vi "testAESEncryptDecrypt-ECB-256.vi"(8 "error in (no error)":errorcluster, 11 "TestCase in":refnum<class "TestAES.lvclass">) -> (0 "error out":errorcluster, 3 "TestCase out":refnum<class "TestAES.lvclass">)   [LabVIEW 2021, in "TestAES.lvclass"]
uses:
  TestAES.lvclass
  C:/Program Files (x86)/National Instruments/LabVIEW 2021/vi.lib/addons/_JKI Toolkits/VI Tester/TestCase.llb/TestCase.lvclass
  TestAES.lvclass/TestAES.ctl
  <vilib>/addons/_JKI Toolkits/VI Tester/TestCase.llb/TestCase.lvclass
  Symmetric Encryption/dotNET Crypto Symmetric Encryption.lvlib
  <vilib>/Wiresmith Technology/VITAC (VI Tester Advanced Comparisons)/VITAC.lvlib
  C:/LabVIEW Working Directory/labview-keystore/Unit Tests/TestAES/TestAES.lvclass
panel:
  out "Plaintext in (hex)":string="Hello, World!"
  out "Key (hex)":string="01234567890"
  out "Expected plaintext (hex)":string
  out "Actual plaintext out (hex)":string
  out "Expected plaintext":string
  out "Plaintext in":string="Hello, World!"
  out "Actual plaintext out":string
  out "Key":string="01234567890"
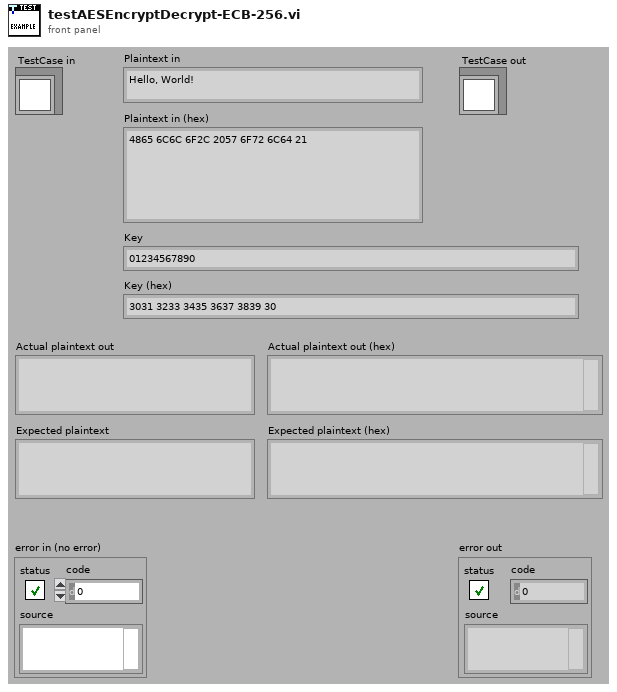
[diagram p1: front panel]
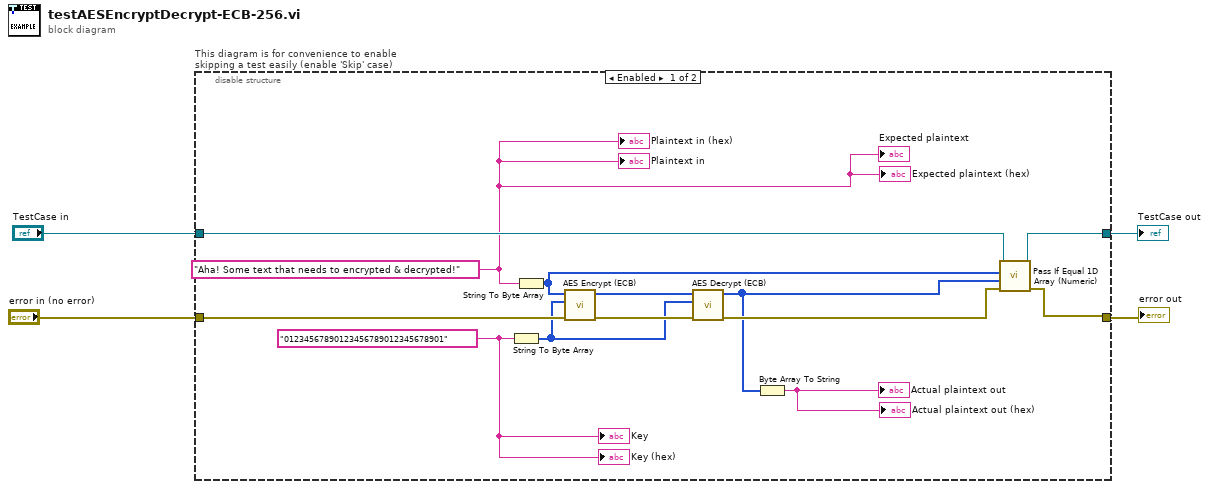
[diagram p0: block diagram]
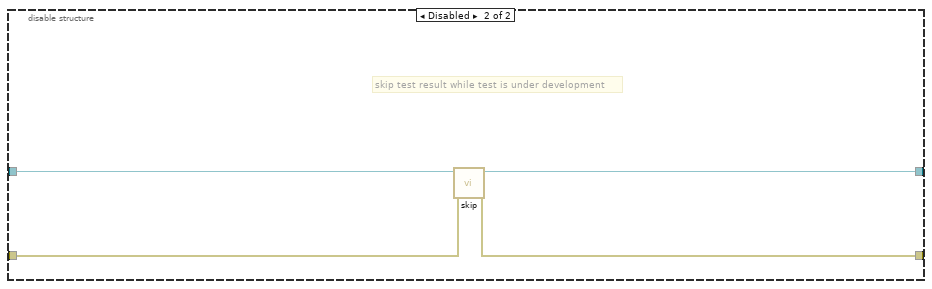
[diagram p2: hidden frame]
diagram:
  n1 = disable-structure "This diagram is for convenience to enable skipping a test easily (enable 'Skip' case)" shown="Enabled" {
    disable-tunnel: "TestCase in" -> [w17 w21]
    disable-tunnel: [w16 w19] -> w1
    disable-tunnel: [w15 w20] -> w3
    disable-tunnel: "error in (no error)" -> [w14 w18]
    frame Enabled {
      w10 = "01234567890123456789012345678901" ("Key")
      w6 = "Aha! Some text that needs to encrypted & decrypted!" ("Plaintext in")
      n2 = String To Byte Array(string=w10) -> (unsigned byte array=w9:u8[])
      n3 = String To Byte Array(string=w6) -> (unsigned byte array=w5:u8[])
      n4 = call "AES Encrypt (ECB).vi"("error in (no error)"=w14, "Key"=w9, "Raw data in"=w5) -> ("error out"=w13:errorcluster, "Encrypted data out"=w11:u8[])  [unwired: 7 in]
      n5 = call "AES Decrypt (ECB).vi"("error in (no error)"=w13, "Key"=w9, "Encrypted data in"=w11) -> ("error out"=w12:errorcluster, "Raw data out"=w7:u8[])  [unwired: 7 in]
      n6 = Byte Array To String(unsigned byte array=w7) -> (string=→"Actual plaintext out" →"Actual plaintext out (hex)":string)
      n7 = call <vilib>:"Pass If Equal 1D Array (Numeric).vi"("error in (no error)"=w12, "actual"=w7, "expected"=w5, "TestCase in"=w17) -> ("error out"=w15:errorcluster, "TestCase out"=w16:refnum<class "TestAES.lvclass">)  [unwired: 6 in]
      "Key" <- w10
      "Plaintext in" <- w6
      "Expected plaintext" <- w6
      "Expected plaintext (hex)" <- w6
      "Key (hex)" <- w10
      "Plaintext in (hex)" <- w6
    }
    frame Disabled {
      # "skip test result while test is under development"
      n8 = call <vilib>:"skip.vi"("error in (no error)"=w18, "TestCase in"=w21) -> ("error out"=w20:errorcluster, "TestCase out"=w19:refnum<class "TestAES.lvclass">)  [unwired: 8 in]
    }
  }
  "error out" <- w3
  "TestCase out" <- w1
